vi "Vector_Dot.vi"(9 "Input Vector 2":T1, 11 "Input Vector 1":T1) -> (3 "dot product":dbl)   [LabVIEW 2019, in "Trajectory_Library.lvlib"]
doc: "Calculate the dot product of two vectors\n\nInputs:\n -- InputVector 1 -- Input vector 1\n -- InputVector 2 -- Input vector 2. This vector must have at least as many rows as vector 1.\n\nOutputs:\n -- Dot Product -- Calculated vector dot product."
uses:
  <vilib>/Analysis/Matrix/Datatypes/RealMatrix.ctl
  Trajectory_Library.lvlib
  <vilib>/Analysis/Matrix/NI_Matrix.lvlib
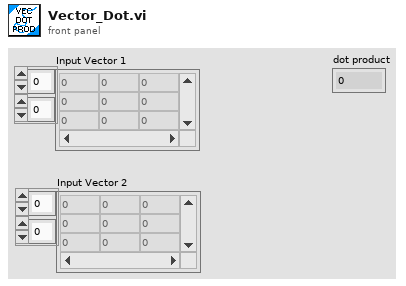
[diagram p1: front panel]
types:
  T1 = typedef "NI_Matrix.lvlib/RealMatrix.ctl" = dbl[][]
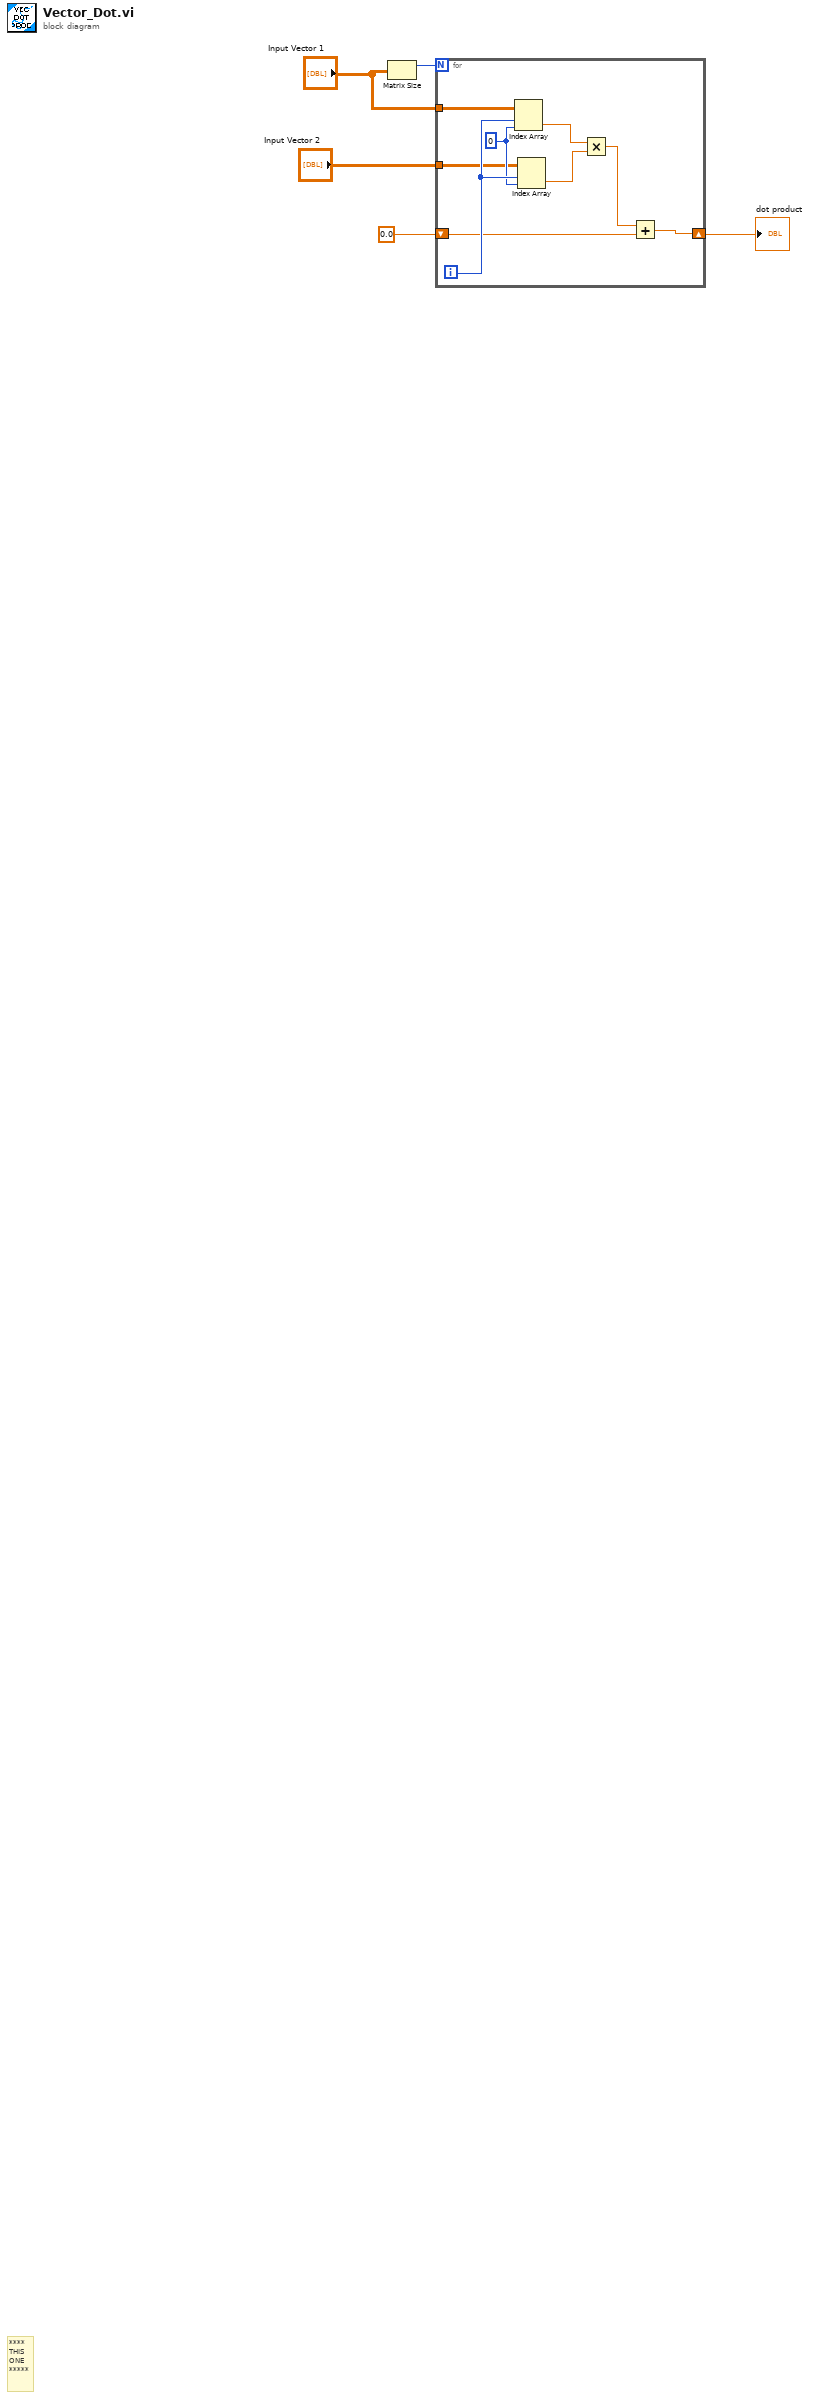
[diagram p0: block diagram]
diagram:
  # "****\nTHIS\nONE\n*****"
  n1 = Matrix Size(0:"Input Vector 1") -> (1:w5:i32)  [unwired: 1 out]
  n2 = for {
    N: w5 -> [_]
    tunnel: "Input Vector 1" -> [w11]
    tunnel: "Input Vector 2" -> [w12]
    shift-right: [w6] -> w1
    shift-left: 0.0 -> [w7]
    i -> [w14]
    w13 = 0 ("index (col)")
    n3 = Index Array(array=w11, index (row)=w14, index (col)=w13) -> (element=w10:dbl)
    n4 = Index Array(array=w12, index (row)=w14, index (col)=w13) -> (element=w9:dbl)
    n5 = Multiply(x=w10, y=w9) -> (x*y=w8:dbl)
    n6 = Add(x=w8, y=w7) -> (x+y=w6:dbl)
  }
  "dot product" <- w1
